vi "LTC1257-DAC.vi"() -> ()   [LabVIEW 2014]
uses:
  <vilib>/MakerHub/LINX/Public/Peripherals/SPI/SPI CS Config.ctl
  <vilib>/MakerHub/LINX/Private/Type Defs/Peripherals/SPI/SPI CS Logic Level.ctl
  <vilib>/MakerHub/LINX/Private/Type Defs/Peripherals/SPI/SPI Configuration.ctl
  <vilib>/MakerHub/LINX/Private/Type Defs/Peripherals/SPI/SPI Bit Order.ctl
  <vilib>/MakerHub/LINX/Private/Type Defs/Peripherals/SPI/SPI Mode.ctl
  <vilib>/MakerHub/LINX/Public/Peripherals/SPI/SPI Write Read 1 Frame.vi
  <vilib>/MakerHub/LINX/Public/Peripherals/SPI/SPI Write Read N Frames.vi
  <vilib>/MakerHub/LINX/Private/Local IO/LinxSpiWriteRead.vi
  <vilib>/MakerHub/LINX/Public/Utilities/Check Channel.vi
  <vilib>/MakerHub/LINX/Public/Utilities/Open Serial.vi
  <vilib>/MakerHub/LINX/Private/Utilties/Generate Error.vi
  <vilib>/MakerHub/LINX/LMH-LINX.lvlib
panel:
  in  "DAC Voltage (0-4095)":u16
  in  "stop":bool
  out "Actual Clock Frequency":u32
  out "DAC Voltage Readout":u16
  out "Error Out":errorcluster
  in  "CS Configuration":T1={"CS Channel"=9, "CS Logic Level"=enum."Active High"}
  out "Device Name":string
  in  "Serial Port":refnum<visa-resource-name>="N/A"
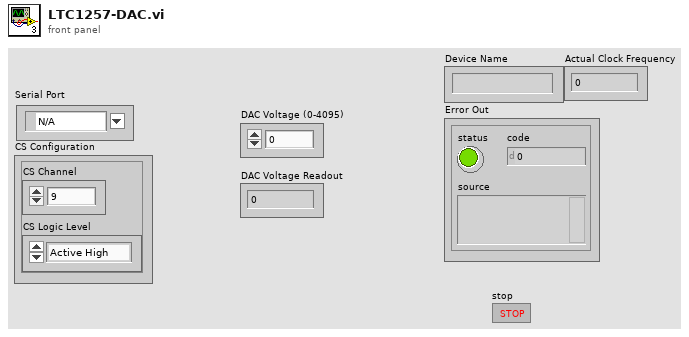
[diagram p1: front panel]
types:
  T1 = typedef "LMH-LINX.lvlib/SPI CS Config.ctl" = cluster{"CS Channel":u8, "CS Logic Level":T2}
  T2 = typedef "LMH-LINX.lvlib/SPI CS Logic Level.ctl" = enum8{"Active Low", "Active High"}
  T3 = typedef "LMH-LINX.lvlib/SPI Configuration.ctl" = cluster{"Clock Frequency":u32, "Bit Order":T4, "SPI Mode":T5}
  T4 = typedef "LMH-LINX.lvlib/SPI Bit Order.ctl" = enum8{"LSb First", "MSb First"}
  T5 = typedef "LMH-LINX.lvlib/SPI Mode.ctl" = enum8{"Mode 0", "Mode 1", "Mode 2", "Mode 3"}
  T6 = typedef "LMH-LINX.lvlib/LINX Ref.ctl" = cluster{"IO":T7, "Interface":T8, "LINX Device Config":T9}
  T7 = typedef "LMH-LINX.lvlib/Platform.ctl" = enum16{"Remote", "Local"}
  T8 = typedef "LMH-LINX.lvlib/Interface.ctl" = enum16{"Serial", "TCP"}
  T9 = typedef "LMH-LINX.lvlib/Device.lvlib/LINX Device Config.ctl" = cluster{"Interface":T8, "COM Port":refnum<visa-resource-name>, "TCP Configuration":T10, "Device Family":u8, "Device ID":u8, "Device Name":string, "TCP Ref":refnum<k5>, "Channels":T11}
  T10 = typedef "LMH-LINX.lvlib/Device.lvlib/TCP Config.ctl" = cluster{"IP Address":string, "Port":u16}
  T11 = typedef "LMH-LINX.lvlib/Channels.ctl" = cluster{"DI":u8[], "DO":u8[], "AI":u8[], "AO":u8[], "PWM":u8[], "QE":u8[], "UART":u8[], "I2C 2":u8[], "SPI":u8[], "CAN":u8[], "Servo":u8[], "AI Ref (V)":dbl, "AI Resolution (Bits)":u8, "AO Ref (V)":dbl, "AO Resolution (Bits)":u8}
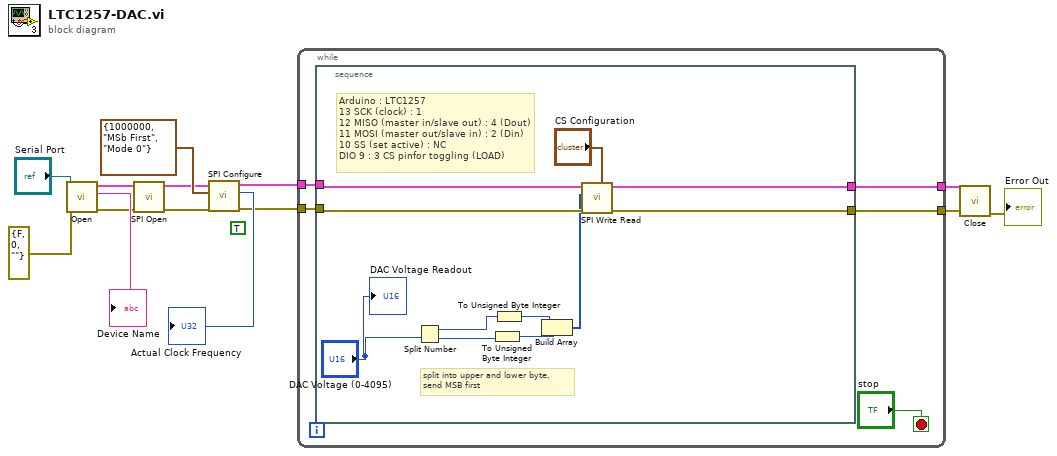
[diagram p0: block diagram]
diagram:
  (unwired) TRUE ("Output Value")
  n1 = call-poly <vilib>:"Open.vi"("Error In"=errorcluster {"status"=FALSE, "code"=0, "source"=""}, "Serial Port"="Serial Port") -> ("Error Out"=w10:errorcluster, "Device Name"=→"Device Name":string, "LINX Resource"=w11:T6)  [unwired: 7 in]
  n2 = call <vilib>:"SPI Open.vi"("Error In"=w10, "LINX Resource"=w11) -> ("Error Out"=w9:errorcluster, "LINX Resource"=w5:T6)  [unwired: 8 in]
  n3 = call <vilib>:"SPI Configure.vi"("Error In"=w9, "SPI Configuration"=T3 {"Clock Frequency"=1000000, "Bit Order"=enum."MSb First", "SPI Mode"=enum."Mode 0"}, "LINX Resource"=w5) -> ("Error Out"=w2:errorcluster, "Actual Clock Frequency"=→"Actual Clock Frequency":u32, "LINX Resource"=w3:T6)  [unwired: 6 in]
  n4 = while {
    tunnel: w3 -> [w16]
    tunnel: w2 -> [w19]
    tunnel: [w15] -> w1
    tunnel: [w17] -> w4
    stop <- "stop" stop-if-true
    n5 = stacked-sequence {
      tunnel: w19 -> [w30]
      tunnel: [w23] -> w17
      tunnel: w16 -> [w21]
      tunnel: [w20] -> w15
      frame #0 {
        # "Arduino : LTC1257\n13 SCK (clock) : 1\n12 MISO (master in/slave out) : 4 (Dout)\n11 MOSI (master out/slave in) : 2 (Din)\n10 SS (set active) : NC\nDIO 9 : 3 CS pinfor toggling (LOAD)"
        # "split into upper and lower byte,\nsend MSB first"
        n6 = Split Number(x="DAC Voltage (0-4095)") -> (hi(x)=w29:u8, lo(x)=w28:u8)
        n7 = To Unsigned Byte Integer(number=w28) -> (unsigned 8bit integer=w25:u8)
        n8 = To Unsigned Byte Integer(number=w29) -> (unsigned 8bit integer=w26:u8)
        n9 = Build Array(w26, w25) -> (w27:u8[])
        n10 = call-poly <vilib>:"SPI Write Read.vi"("CS Configuration"="CS Configuration", "Error In"=w30, "Data"=w27, "LINX Resource"=w21) -> ("Error Out"=w23:errorcluster, "LINX Resource"=w20:T6)  [unwired: 5 in, 1 out]
        "DAC Voltage Readout" <- "DAC Voltage (0-4095)"
      }
    }
  }
  n11 = call <vilib>:"Close.vi"("Error In"=w4, "LINX Resource"=w1) -> ("Error Out"=→"Error Out":errorcluster)  [unwired: 9 in]
